vi "Populate List Box.vi"(7 "Listbox Ref":refnum<vi>, 8 "Error In":errorcluster, 11 "Dependecy Config":T1) -> (0 "Error Out":errorcluster, 3 "Dependecy Config":T1)   [LabVIEW 2014, in "LMH-Toolbox.lvlib" / "LMH-Installer Tools.lvlib"]
uses:
  <vilib>/MakerHub/Toolbox/Private/Installer Tools/LMH-Installer Tools.lvlib
  <vilib>/MakerHub/Toolbox/Private/Installer Tools/Private/Type Defs/Dependency Config.ctl
  <vilib>/MakerHub/Toolbox/Private/Installer Tools/Private/Type Defs/Dependecy.ctl
  <vilib>/MakerHub/Toolbox/Private/Web/Type Defs/Download Task.ctl
  <vilib>/picture/picture.llb/imagedata.ctl
  <vilib>/MakerHub/Toolbox/Private/Web/LMH-Web.lvlib
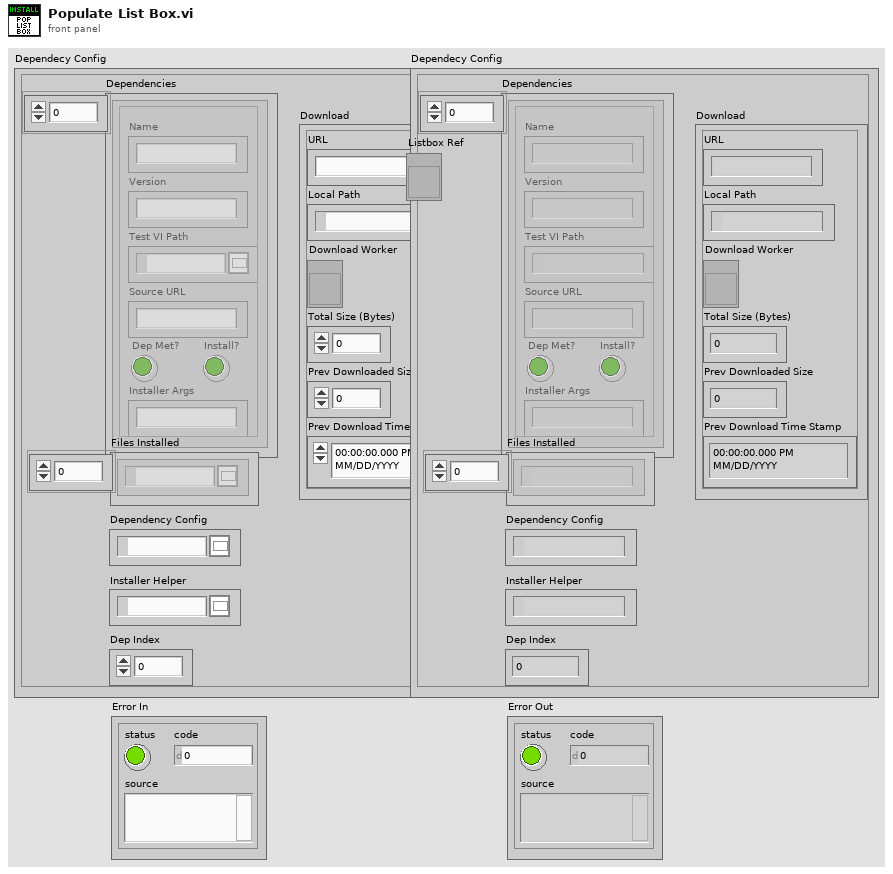
[diagram p1: front panel]
types:
  T1 = typedef "LMH-Toolbox.lvlib/LMH-Installer Tools.lvlib/Dependency Config.ctl" = cluster{"Dependencies":T2[], "Files Installed":path[], "Dependency Config":path, "Installer Helper":path, "Dep Index":i32, "Download":T3}
  T2 = typedef "LMH-Toolbox.lvlib/LMH-Installer Tools.lvlib/Dependecy.ctl" = cluster{"Name":string, "Version":string, "Test VI Path":path, "Source URL":string, "Dep Met?":bool, "Install?":bool, "Installer Args":string}
  T3 = typedef "LMH-Toolbox.lvlib/LMH-Web.lvlib/Download Task.ctl" = cluster{"URL":string, "Local Path":path, "Download Worker":refnum<vi>, "Total Size (Bytes)":u64, "Prev Downloaded Size":u64, "Prev Download Time Stamp":timestamp}
  T4 = typedef "imagedata.ctl" = cluster{"image type":i32, "image depth":i32, "image":u8[], "mask":u8[], "colors":u32[], "Rectangle":cluster{"left":i16, "top":i16, "right":i16, "bottom":i16}}
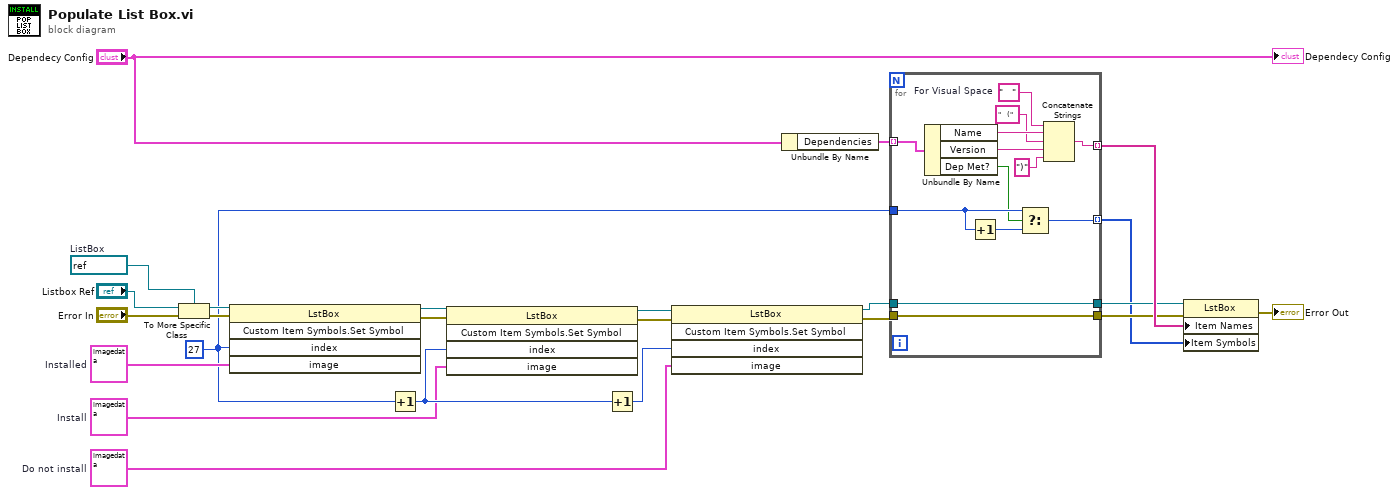
[diagram p0: block diagram]
diagram:
  w2 = 27 ("Index")
  w3 = T4 {"image type"=0, "image depth"=32, "image"=[0, 255, 255, 255, 0, 255, 255, 255, 0, 255, 255, 255, 255, 128, 0, 0, 255, 128, 0, 0, 255, 128, 0, 0, 0, 255, 255, 255, 0, 255, 255, 255, 0, 255, 255, 255, 0, 255, 255, 255, 255, 128, 0, 0, 255, 128, 0, 0, 255, 128, 0, 0, 0, 255, 255, 255, 0, 255, 255, 255, 0, 255, 255, 255, 0, 255, 255, 255, 0, 255, 255, 255, 0, 255, 255, 255, 0, 255, 255, 255, 255, 128, 0, 0, 255, 128, 0, 0, 255, 128, 0, 0, 0, 255, 255, 255, 0, 255, 255, 255, 255, 128, 0, 0, 255, 128, 0, 0, 255, 128, 0, 0, 0, 255, 255, 255, 0, 255, 255, 255, 0, 255, 255, 255, 0, 255, 255, 255, 0, 255, 255, 255, 0, 255, 255, 255, 0, 255, 255, 255, 0, 255, 255, 255, 0, 255, 255, 255, 255, 128, 0, 0, 255, 128, 0, 0, 255, 128, 0, 0, 255, 128, 0, 0, 255, 128, 0, 0, 255, 128, 0, 0, 0, 255, 255, 255, 0, 255, 255, 255, 0, 255, 255, 255, 0, 255, 255, 255, 0, 255, 255, 255, 0, 255, 255, 255, 0, 255, 255, 255, 0, 255, 255, 255, 0, 255, 255, 255, 0, 255, 255, 255, 0, 255, 255, 255, 255, 128, 0, 0, 255, 128, 0, 0, 255, 128, 0, 0, 255, 128, 0, 0, 0, 255, 255, 255, 0, 255, 255, 255, 0, 255, 255, 255, 0, 255, 255, 255, 0, 255, 255, 255, 0, 255, 255, 255, 0, 255, 255, 255, 0, 255, 255, 255, 0, 255, 255, 255, 0, 255, 255, 255, 0, 255, 255, 255, 0, 255, 255, 255, 0, 255, 255, 255, 255, 128, 0, 0, 255, 128, 0, 0, 0, 255, 255, 255, 0, 255, 255, 255, 0, 255, 255, 255, 0, 255, 255, 255, 0, 255, 255, 255, 0, 255, 255, 255, 0, 255, 255, 255, 0, 255, 255, 255, 0, 255, 255, 255, 0, 255, 255, 255, 0, 255, 255, 255, 0, 255, 255, 255, 0, 255, 255, 255, 255, 128, 0, 0, 255, 128, 0, 0, 255, 128, 0, 0, 255, 128, 0, 0, 0, 255, 255, 255, 0, 255, 255, 255, 0, 255, 255, 255, 0, 255, 255, 255, 0, 255, 255, 255, 0, 255, 255, 255, 0, 255, 255, 255, 0, 255, 255, 255, 255, 134, 134, 134, 255, 134, 134, 134, 255, 134, 134, 134, 255, 128, 0, 0, 255, 128, 0, 0, 255, 128, 0, 0, 255, 128, 0, 0, 255, 128, 0, 0, 255, 128, 0, 0, 255, 134, 134, 134, 255, 134, 134, 134, 255, 134, 134, 134, 255, 134, 134, 134, 0, 255, 255, 255, 0, 255, 255, 255, 255, 134, 134, 134, 255, 192, 192, 192, 255, 192, 192, 192, 255, 128, 0, 0, 255, 128, 0, 0, 255, 128, 0, 0, 255, 192, 192, 192, 255, 192, 192, 192, 255, 128, 0, 0, 255, 128, 0, 0, 255, 128, 0, 0, 255, 192, 192, 192, 255, 192, 192, 192, 255, 76, 76, 76, 255, 0, 0, 0, 255, 134, 134, 134, 255, 255, 255, 255, 255, 255, 255, 255, 255, 128, 0, 0, 255, 128, 0, 0, 255, 128, 0, 0, 255, 255, 255, 255, 255, 255, 255, 255, 255, 255, 255, 255, 255, 255, 255, 255, 255, 128, 0, 0, 255, 128, 0, 0, 255, 128, 0, 0, 255, 119, 119, 119, 255, 76, 76, 76, 255, 0, 0, 0, 255, 134, 134, 134, 255, 255, 255, 255, 255, 231, 231, 214, 255, 192, 192, 192, 255, 192, 192, 192, 255, 192, 192, 192, 255, 192, 192, 192, 255, 192, 192, 192, 255, 192, 192, 192, 255, 153, 255, 0, 255, 0, 255, 0, 255, 0, 153, 0, 255, 204, 204, 153, 255, 119, 119, 119, 255, 76, 76, 76, 255, 0, 0, 0, 255, 134, 134, 134, 255, 255, 255, 255, 255, 204, 204, 153, 255, 204, 204, 153, 255, 204, 204, 153, 255, 204, 204, 153, 255, 204, 204, 153, 255, 204, 204, 153, 255, 204, 204, 153, 255, 204, 204, 153, 255, 204, 204, 153, 255, 204, 204, 153, 255, 204, 204, 153, 255, 119, 119, 119, 255, 76, 76, 76, 255, 0, 0, 0, 255, 134, 134, 134, 255, 134, 134, 134, 255, 134, 134, 134, 255, 134, 134, 134, 255, 134, 134, 134, 255, 134, 134, 134, 255, 134, 134, 134, 255, 134, 134, 134, 255, 134, 134, 134, 255, 134, 134, 134, 255, 134, 134, 134, 255, 134, 134, 134, 255, 134, 134, 134, 255, 134, 134, 134, 255, 0, 0, 0, 0, 255, 255, 255, 0, 255, 255, 255, 255, 0, 0, 0, 255, 0, 0, 0, 255, 0, 0, 0, 255, 0, 0, 0, 255, 0, 0, 0, 255, 0, 0, 0, 255, 0, 0, 0, 255, 0, 0, 0, 255, 0, 0, 0, 255, 0, 0, 0, 255, 0, 0, 0, 255, 0, 0, 0, 255, 0, 0, 0, 0, 255, 255, 255, 0, 255, 255, 255], "mask"=[28, 56, 14, 112, 7, 224, 3, 192, 1, 128, 3, 192, 63, 254, 127, 255, 255, 255, 255, 255, 255, 255, 255, 254, 127, 252], "colors"=[], "Rectangle"={"left"=0, "top"=0, "right"=16, "bottom"=13}}  # Do not install
  w5 = T4 {"image type"=0, "image depth"=32, "image"=[0, 255, 255, 255, 0, 255, 255, 255, 0, 255, 255, 255, 0, 85, 197, 73, 0, 117, 195, 49, 0, 85, 197, 73, 2, 112, 201, 102, 1, 85, 197, 73, 0, 76, 190, 48, 79, 34, 139, 19, 255, 40, 161, 23, 255, 40, 161, 23, 0, 255, 255, 255, 0, 255, 255, 255, 0, 255, 255, 255, 0, 255, 255, 255, 0, 255, 255, 255, 0, 255, 255, 255, 0, 255, 255, 255, 0, 255, 255, 255, 0, 48, 182, 29, 0, 85, 197, 73, 1, 85, 197, 73, 0, 76, 190, 48, 3, 48, 182, 29, 255, 40, 161, 23, 255, 34, 139, 19, 0, 255, 255, 255, 0, 255, 255, 255, 0, 255, 255, 255, 0, 255, 255, 255, 0, 255, 255, 255, 0, 255, 255, 255, 0, 255, 255, 255, 0, 255, 255, 255, 0, 255, 255, 255, 0, 255, 255, 255, 255, 34, 139, 19, 255, 40, 161, 23, 0, 48, 182, 29, 255, 40, 161, 23, 255, 34, 139, 19, 0, 255, 255, 255, 0, 255, 255, 255, 0, 255, 255, 255, 0, 255, 255, 255, 0, 255, 255, 255, 0, 255, 255, 255, 0, 255, 255, 255, 0, 255, 255, 255, 0, 255, 255, 255, 0, 255, 255, 255, 0, 255, 255, 255, 0, 255, 255, 255, 255, 34, 139, 19, 255, 40, 161, 23, 255, 34, 139, 19, 0, 255, 255, 255, 0, 255, 255, 255, 0, 255, 255, 255, 0, 255, 255, 255, 0, 255, 255, 255, 0, 255, 255, 255, 0, 255, 255, 255, 0, 255, 255, 255, 0, 255, 255, 255, 0, 255, 255, 255, 0, 255, 255, 255, 0, 255, 255, 255, 0, 255, 255, 255, 0, 255, 255, 255, 255, 34, 139, 19, 0, 255, 255, 255, 0, 255, 255, 255, 0, 255, 255, 255, 0, 255, 255, 255, 0, 255, 255, 255, 0, 255, 255, 255, 0, 255, 255, 255, 0, 255, 255, 255, 0, 255, 255, 255, 0, 255, 255, 255, 255, 134, 134, 134, 255, 134, 134, 134, 255, 134, 134, 134, 255, 134, 134, 134, 255, 134, 134, 134, 255, 134, 134, 134, 255, 134, 134, 134, 255, 134, 134, 134, 255, 134, 134, 134, 255, 134, 134, 134, 255, 134, 134, 134, 255, 134, 134, 134, 255, 134, 134, 134, 0, 255, 255, 255, 0, 255, 255, 255, 255, 134, 134, 134, 255, 192, 192, 192, 255, 192, 192, 192, 255, 192, 192, 192, 255, 192, 192, 192, 255, 192, 192, 192, 255, 192, 192, 192, 255, 192, 192, 192, 255, 192, 192, 192, 255, 192, 192, 192, 255, 192, 192, 192, 255, 192, 192, 192, 255, 192, 192, 192, 255, 76, 76, 76, 255, 0, 0, 0, 255, 134, 134, 134, 255, 255, 255, 255, 255, 255, 255, 255, 255, 255, 255, 255, 255, 255, 255, 255, 255, 255, 255, 255, 255, 255, 255, 255, 255, 255, 255, 255, 255, 255, 255, 255, 255, 255, 255, 255, 255, 255, 255, 255, 255, 255, 255, 255, 255, 255, 255, 255, 255, 119, 119, 119, 255, 76, 76, 76, 255, 0, 0, 0, 255, 134, 134, 134, 255, 255, 255, 255, 255, 231, 231, 214, 255, 192, 192, 192, 255, 192, 192, 192, 255, 192, 192, 192, 255, 192, 192, 192, 255, 192, 192, 192, 255, 192, 192, 192, 255, 153, 255, 0, 255, 0, 255, 0, 255, 0, 153, 0, 255, 204, 204, 153, 255, 119, 119, 119, 255, 76, 76, 76, 255, 0, 0, 0, 255, 134, 134, 134, 255, 255, 255, 255, 255, 204, 204, 153, 255, 204, 204, 153, 255, 204, 204, 153, 255, 204, 204, 153, 255, 204, 204, 153, 255, 204, 204, 153, 255, 204, 204, 153, 255, 204, 204, 153, 255, 204, 204, 153, 255, 204, 204, 153, 255, 204, 204, 153, 255, 119, 119, 119, 255, 76, 76, 76, 255, 0, 0, 0, 255, 134, 134, 134, 255, 134, 134, 134, 255, 134, 134, 134, 255, 134, 134, 134, 255, 134, 134, 134, 255, 134, 134, 134, 255, 134, 134, 134, 255, 134, 134, 134, 255, 134, 134, 134, 255, 134, 134, 134, 255, 134, 134, 134, 255, 134, 134, 134, 255, 134, 134, 134, 255, 134, 134, 134, 255, 0, 0, 0, 0, 255, 255, 255, 0, 255, 255, 255, 255, 0, 0, 0, 255, 0, 0, 0, 255, 0, 0, 0, 255, 0, 0, 0, 255, 0, 0, 0, 255, 0, 0, 0, 255, 0, 0, 0, 255, 0, 0, 0, 255, 0, 0, 0, 255, 0, 0, 0, 255, 0, 0, 0, 255, 0, 0, 0, 255, 0, 0, 0, 0, 255, 255, 255, 0, 255, 255, 255], "mask"=[0, 48, 0, 96, 6, 192, 3, 128, 1, 0, 63, 254, 127, 255, 255, 255, 255, 255, 255, 255, 255, 254, 127, 252], "colors"=[], "Rectangle"={"left"=0, "top"=0, "right"=16, "bottom"=12}}  # Installed
  w4 = T4 {"image type"=0, "image depth"=32, "image"=array[960 elements], "mask"=[7, 192, 7, 192, 7, 192, 31, 240, 15, 224, 7, 192, 3, 128, 1, 0, 63, 254, 127, 255, 255, 255, 255, 255, 255, 255, 255, 254, 127, 252], "colors"=[], "Rectangle"={"left"=0, "top"=0, "right"=16, "bottom"=15}}  # Install
  w20 = refnum<vi> refnum  # ListBox
  n1 = To More Specific Class(target class=w20, reference="Listbox Ref", error in="Error In") -> (specific class reference=w15:refnum<vi>, error out=w13:errorcluster)
  n2 = invoke class="LstBox" method="Custom Item Symbols.Set Symbol"(reference=w15, error in=w13, "index"=w2, "image"=w5) -> (reference out=w12:refnum<vi>, error out=w14:errorcluster)  [unwired: 1 in, 3 out]
  n3 = Increment(x=w2) -> (x+1=w6:i32)
  n4 = invoke class="LstBox" method="Custom Item Symbols.Set Symbol"(reference=w12, error in=w14, "index"=w6, "image"=w4) -> (reference out=w9:refnum<vi>, error out=w11:errorcluster)  [unwired: 1 in, 3 out]
  n5 = Increment(x=w6) -> (x+1=w7:i32)
  n6 = invoke class="LstBox" method="Custom Item Symbols.Set Symbol"(reference=w9, error in=w11, "index"=w7, "image"=w3) -> (reference out=w8:refnum<vi>, error out=w10:errorcluster)  [unwired: 1 in, 3 out]
  n7 = Unbundle By Name("Dependecy Config") -> ("Dependencies"=w23:T2[])
  n8 = for {
    tunnel: w23 -> [w37] mode=indexing
    tunnel: w10 -> [w32]
    tunnel: w8 -> [w31]
    tunnel: [w33] -> w19 mode=indexing
    tunnel: [w32] -> w18
    tunnel: [w31] -> w17
    tunnel: w2 -> [w28]
    tunnel: [w26] -> w1 mode=indexing
    w25 = "   "  # For Visual Space
    n9 = Unbundle By Name(w37) -> ("Name"=w36:string, "Version"=w34:string, "Dep Met?"=w27:bool)
    n10 = Increment(x=w28) -> (x+1=w29:i32)
    n11 = Select(t=w28, s=w27, f=w29) -> (s? t:f=w26:i32)
    n12 = Concatenate Strings(w25, w36, "   (" ("string"), w34, ")" ("string")) -> (w33:string)
  }
  n13 = property class="LstBox"(reference=w17, error in=w18, "Item Names"=w19, "Item Symbols"=w1) -> (error out=→"Error Out":errorcluster)  [unwired: 1 out]
  "Dependecy Config" <- "Dependecy Config"
